vi "shift.vi"(6 "shift":bool, 7 "using":enum16{"position", "time"}(ring), 9 "delta_x":dbl, 10 "threshold":dbl, 11 "txv IN":T1) -> (3 "txv OUT":T1)   [LabVIEW 2017, in "wf.lvlib"]
uses:
  wf.lvlib
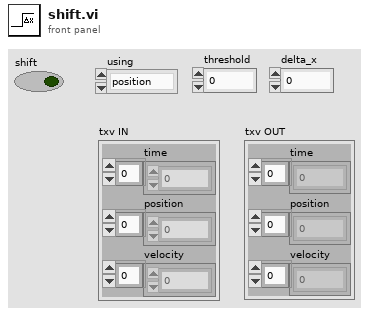
[diagram p1: front panel]
types:
  T1 = cluster{"time":dbl[], "position":dbl[], "velocity":dbl[]}
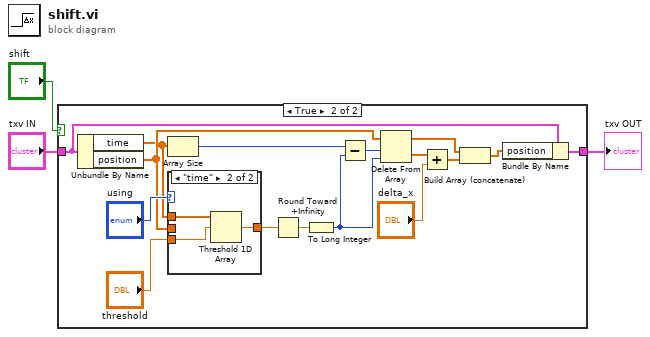
[diagram p0: block diagram]
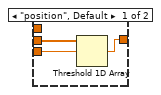
[diagram p3: hidden frame]
diagram:
  n1 = case shown="True" "shift" {
    tunnel: "txv IN" -> [w4 w7]
    tunnel: [w4 w5] -> w3
    frame False {
    }
    frame True {
      n2 = Unbundle By Name(w7) -> ("time"=w8:dbl[], "position"=w18:dbl[])
      n3 = Array Size(array=w8) -> (size(s)=w15:i32)
      n4 = case shown="\"time\"" "using" {
        tunnel: w8 -> [_ w25]
        tunnel: "threshold" -> [w22 w26]
        tunnel: w18 -> [w23 _]
        tunnel: [w21 w24] -> w14
        frame "position", Default {
          n5 = Threshold 1D Array(2:w22, 3:w23) -> (0:w21:dbl)  [unwired: 1 in]
        }
        frame "time" {
          n6 = Threshold 1D Array(2:w26, 3:w25) -> (0:w24:dbl)  [unwired: 1 in]
        }
      }
      n7 = Round Toward +Infinity(x=w14) -> (ceil(x): smallest int >= x=w10:dbl)
      n8 = To Long Integer(number=w10) -> (32bit integer=w16:i32)
      n9 = Subtract(x=w15, y=w16) -> (x-y=w9:i32)
      n10 = Delete From Array(array=w18, length=w9, index=w16) -> (deleted portion=w11:dbl[], array with subset deleted=w13:dbl[])
      n11 = Add(x=w11, y="delta_x") -> (x+y=w12:dbl[])
      n12 = Build Array (concatenate)(w13, w12) -> (w6:dbl[])
      n13 = Bundle By Name(cluster=w7, "position"=w6) -> (w5:T1)
    }
  }
  "txv OUT" <- w3
